vi "Drive Process.vi"(0 "error in":errorcluster) -> ()   [LabVIEW 2013]
uses:
  Drive Global Data.vi
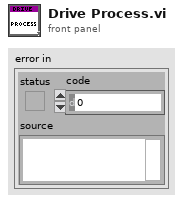
[diagram p1: front panel]
types:
  T1 = cluster{"Y":dbl, "X":dbl, "Left Encoder":dbl, "Right Encoder":dbl}
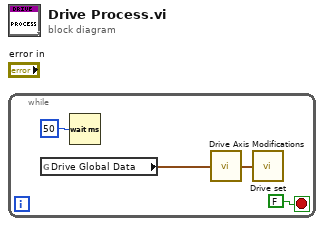
[diagram p0: block diagram]
diagram:
  n1 = while {
    stop <- FALSE stop-if-true
    n2 = global read "Drive Global Data.vi" "Drive Global Data"() -> (w1:T1)
    n3 = Wait (ms)(milliseconds to wait=u32 50) -> ()  [unwired: 1 out]
    n4 = call "Drive Axis Modifications.vi"("Drive Global Data In"=w1) -> ("Drive Global Data Out"=w3:T1)
    n5 = call "Drive set.vi"("Drive Global Data"=w3) -> ()
  }
